vi "Open_DSP.vi"(8 "error in":errorcluster, 10 "Byte count":u32=100, 11 "VISA":refnum<visa-resource-name>) -> (0 "error out":errorcluster, 2 "read buffer":string, 3 "VISA out":refnum<visa-resource-name>)   [LabVIEW 2019]
uses:
  <vilib>/Instr/_visa.llb/VISA Open Access Mode.ctl
panel:
  out "길이":i32
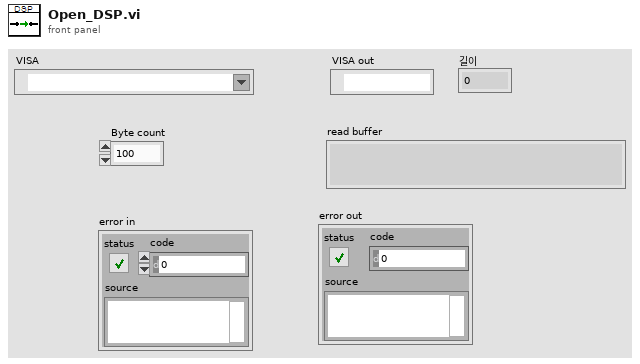
[diagram p1: front panel]
types:
  T1 = typedef "VISA Open Access Mode.ctl" = u32
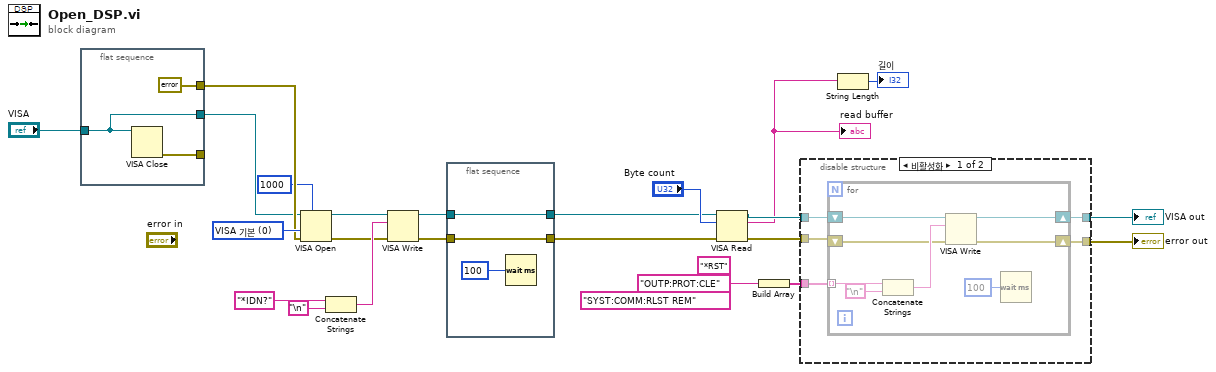
[diagram p0: block diagram]
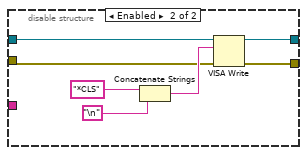
[diagram p2: hidden frame]
diagram:
  (unwired) "*RST" ("Command")
  (unwired) "SYST:COMM:RLST REM"
  w16 = T1 0 items=["VISA 기본"=0, "배타적인 잠금"=1, "설정된 셋팅 로드"=4] ("Access Mode")
  n1 = flat-sequence {
    tunnel: "VISA" -> [w24]
    tunnel: [w26] -> _
    tunnel: [errorcluster {"status"=FALSE, "code"=0, "source"=""} ("에러 입력(에러 없음)")] -> w3
    tunnel: [w24] -> w2
    frame #0 {
      n2 = VISA Close(VISA resource name=w24) -> (error out=w26:errorcluster)  [unwired: 1 in]
    }
  }
  n3 = VISA Open(timeout (0)=u32 1000 ("VISA Open timeout (0)"), access mode=w16, error in (no error)=w3, VISA resource name=w2) -> (VISA resource name=w15:refnum<visa-resource-name>, error out=w13:errorcluster)  [unwired: 1 in]
  n4 = Concatenate Strings("*IDN?" ("Command"), "\n") -> (w18:string)
  n5 = VISA Write(VISA resource name=w15, write buffer=w18, error in (no error)=w13) -> (VISA resource name out=w22:refnum<visa-resource-name>, error out=w21:errorcluster)  [unwired: 1 out]
  n6 = flat-sequence {
    tunnel: w22 -> [w29]
    tunnel: w21 -> [w28]
    tunnel: [w29] -> w20
    tunnel: [w28] -> w19
    frame #0 {
      n7 = Wait (ms)(milliseconds to wait=u32 100 ("대기 시간 (ms)")) -> ()  [unwired: 1 out]
    }
  }
  n8 = VISA Read(VISA resource name=w20, byte count="Byte count", error in (no error)=w19) -> (VISA resource name out=w12:refnum<visa-resource-name>, read buffer=w6:string, error out=w11:errorcluster)  [unwired: 1 out]
  "read buffer" <- w6
  n9 = Build Array("OUTP:PROT:CLE" ("Command")) -> (w7:string[])
  n10 = disable-structure shown="비활성화" {
    disable-tunnel: w12 -> [w34 w47]
    disable-tunnel: w11 -> [w33 w43]
    disable-tunnel: [w32 w46] -> w10
    disable-tunnel: [w31 w45] -> w9
    disable-tunnel: w7 -> [w30 _]
    frame Disabled {
      n11 = for {
        shift-right: [w38] -> w32
        shift-left: w34 -> [w40]
        shift-right: [w37] -> w31
        shift-left: w33 -> [w39]
        tunnel: w30 -> [w36] mode=indexing
        n12 = Concatenate Strings(w36, "\n") -> (w42:string)
        n13 = VISA Write(VISA resource name=w40, write buffer=w42, error in (no error)=w39) -> (VISA resource name out=w38:refnum<visa-resource-name>, error out=w37:errorcluster)  [unwired: 1 out]
        n14 = Wait (ms)(milliseconds to wait=u32 100) -> ()  [unwired: 1 out]
      }
    }
    frame Enabled {
      n15 = Concatenate Strings("*CLS" ("Command"), "\n") -> (w44:string)
      n16 = VISA Write(VISA resource name=w47, write buffer=w44, error in (no error)=w43) -> (VISA resource name out=w46:refnum<visa-resource-name>, error out=w45:errorcluster)  [unwired: 1 out]
    }
  }
  "VISA out" <- w10
  "error out" <- w9
  n17 = String Length(string=w6) -> (length=→"길이":i32)
